vi "open_matfile.vi"(5 "file_name":string="prova.mat", 7 "error in":errorcluster, 8 "access (0:read/write)":enum16{"read/write", "read-only", "write-only"}(ring), 9 "operation (0:open)":T3(ring), 10 "file path (use dialog)":path) -> (0 "error out":errorcluster, 3 "matFile_info":T1)   [LabVIEW 2018]
uses:
  MatFile_information.ctl
  type_control.ctl
panel:
  out "refnum out":refnum<file>
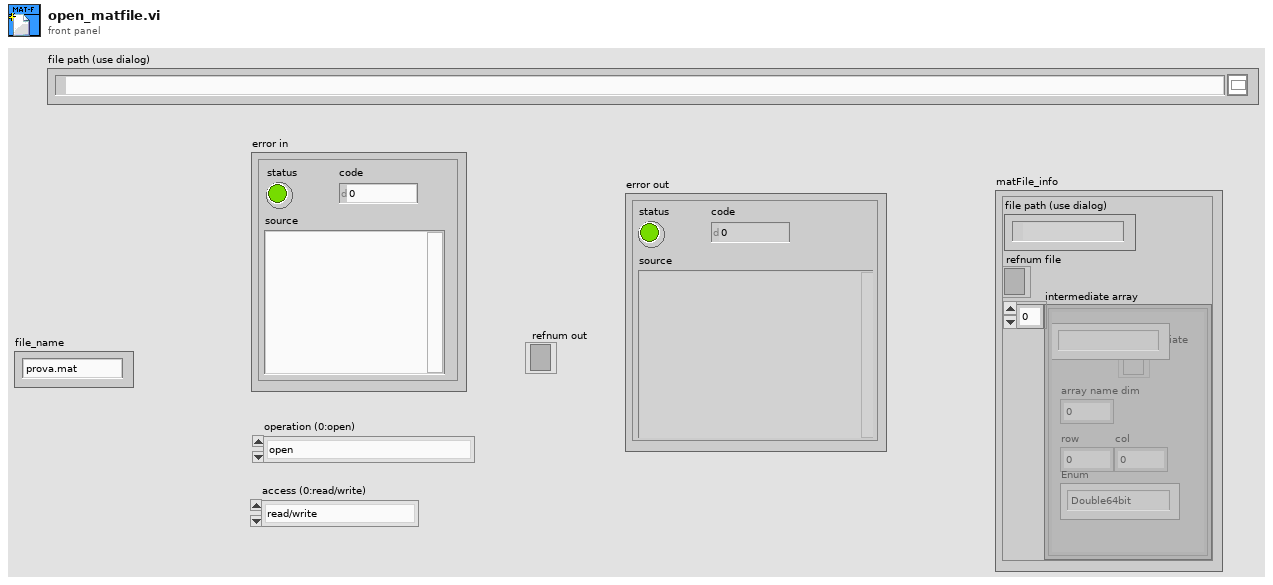
[diagram p1: front panel]
types:
  T1 = typedef "MatFile_information.ctl" = cluster{"file path (use dialog)":path, "refnum file":refnum<file>, "intermediate array":cluster{"intermediate":refnum<file>, "array name dim":i32, "row":i32, "col":i32, "Content":string, "Enum":T2}[]}
  T2 = typedef "type_control.ctl" = enum16{"Int8bit_elem", "Int8bit", "Int64bit_elem", "Int64bit", "Int16bit_elem", "Double64bit_elem", "Int16bit", "Double64bit"}
  T3 = enum16{"open", "replace", "create", "open or create", "replace or create", "replace or create with confirmation"}
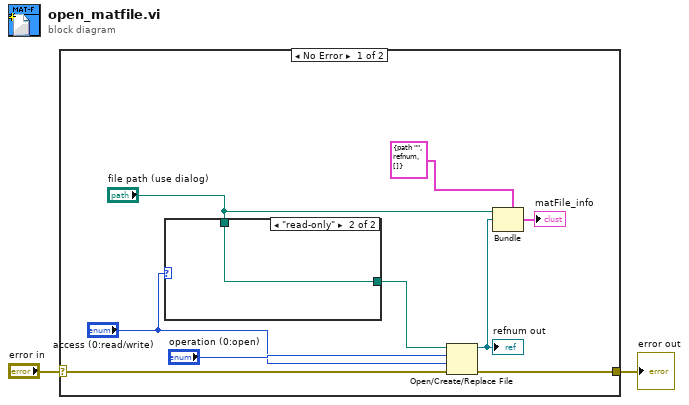
[diagram p0: block diagram]
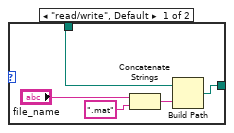
[diagram p2: hidden frame]
diagram:
  n1 = case shown="No Error" "error in" {
    selector: "error in" -> [w10 w18]
    tunnel: [w5 w18] -> w1
    frame No Error {
      n2 = case shown="\"read-only\"" "access (0:read/write)" {
        tunnel: "file path (use dialog)" -> [w13 w17]
        tunnel: [w12 w17] -> w7
        frame "read/write", Default {
          n3 = Concatenate Strings("file_name", ".mat" ("string")) -> (w15:string)
          n4 = Build Path(base path=w13, name or relative path=w15) -> (appended path=w12:path)
        }
        frame "read-only" {
        }
      }
      n5 = Open/Create/Replace File(file path (use dialog)=w7, error in=w10, operation (0:open)="operation (0:open)", access (0:read/write)="access (0:read/write)") -> (refnum out=w6:refnum<file>, error out=w5:errorcluster)  [unwired: 2 in, 1 out]
      "refnum out" <- w6
      n6 = Bundle(cluster=T1 {"file path (use dialog)"=path "", "refnum file"=refnum, "intermediate array"=[]} ("matFile_info"), "file path (use dialog)"="file path (use dialog)", "refnum file"=w6) -> (→"matFile_info":T1)  [unwired: 1 in]
    }
    frame Error {
    }
  }
  "error out" <- w1
